vi "TestAdm_TimerWait.vi"(5 "error in (no error)":errorcluster, 7 "milliseconds to wait":u32) -> (19 "error out":errorcluster)   [LabVIEW 2009]
doc: "Waits for number of milliseconds stated in \"milliseconds to wait\""
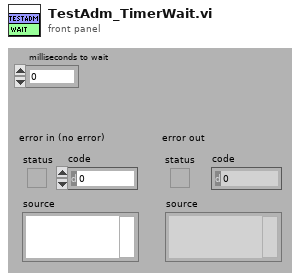
[diagram p1: front panel]
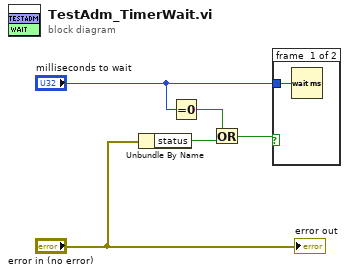
[diagram p0: block diagram]
diagram:
  n1 = Unbundle By Name("error in (no error)") -> ("status"=w4:bool)
  n2 = Equal To 0?(x="milliseconds to wait") -> (x = 0?=w1:bool)
  n3 = Or(x=w1, y=w4) -> (x .or. y?=w3:bool)
  n4 = case shown="False" w3 {
    tunnel: "milliseconds to wait" -> [w6 _]
    frame #0 {
      n5 = Wait (ms)(milliseconds to wait=w6) -> ()  [unwired: 1 out]
    }
    frame #1 {
    }
  }
  "error out" <- "error in (no error)"
